vi "位置显示 ccd2.vi"(8 "error in (no error) 2":errorcluster, 10 "簇":T2, 11 "Image in":T1(plugin-control)) -> (0 "error out":errorcluster caption="错误输出", 1 "下":dbl, 2 "上":dbl, 3 "Image out":T1(plugin-control), 4 "x或y？":bool)   [LabVIEW 2017]
panel:
  out "xia":dbl
  out "shang":dbl
  out "x/y":dbl
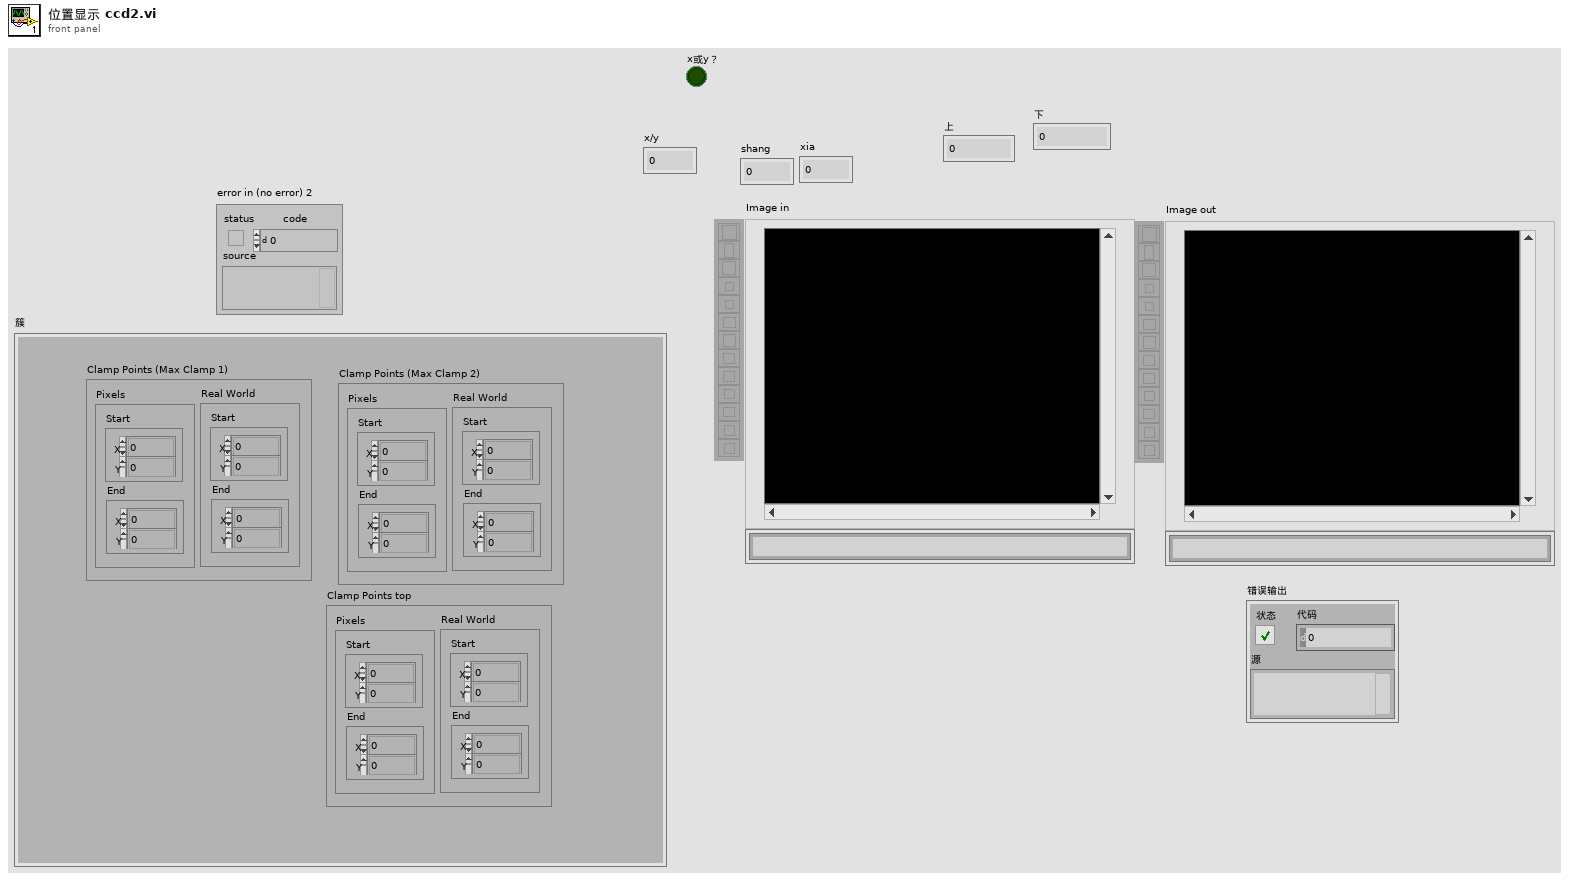
[diagram p1: front panel]
types:
  T1 = typedef "IMAQ Image.ctl" = refnum<image>
  T2 = cluster{"Clamp Points (Max Clamp 1)":cluster{"Pixels ":cluster{"Start":cluster{"X":dbl, "Y":dbl}, "End":cluster{"X":dbl, "Y":dbl}}, "Real World":cluster{"Start":cluster{"X":dbl, "Y":dbl}, "End":cluster{"X":dbl, "Y":dbl}}}, "Clamp Points (Max Clamp 2)":cluster{"Pixels ":cluster{"Start":cluster{"X":dbl, "Y":dbl}, "End":cluster{"X":dbl, "Y":dbl}}, "Real World":cluster{"Start":cluster{"X":dbl, "Y":dbl}, "End":cluster{"X":dbl, "Y":dbl}}}, "Clamp Points top":cluster{"Pixels ":cluster{"Start":cluster{"X":dbl, "Y":dbl}, "End":cluster{"X":dbl, "Y":dbl}}, "Real World":cluster{"Start":cluster{"X":dbl, "Y":dbl}, "End":cluster{"X":dbl, "Y":dbl}}}}
  T3 = cluster{"Pixels ":cluster{"Start":cluster{"X":dbl, "Y":dbl}, "End":cluster{"X":dbl, "Y":dbl}}, "Real World":cluster{"Start":cluster{"X":dbl, "Y":dbl}, "End":cluster{"X":dbl, "Y":dbl}}}
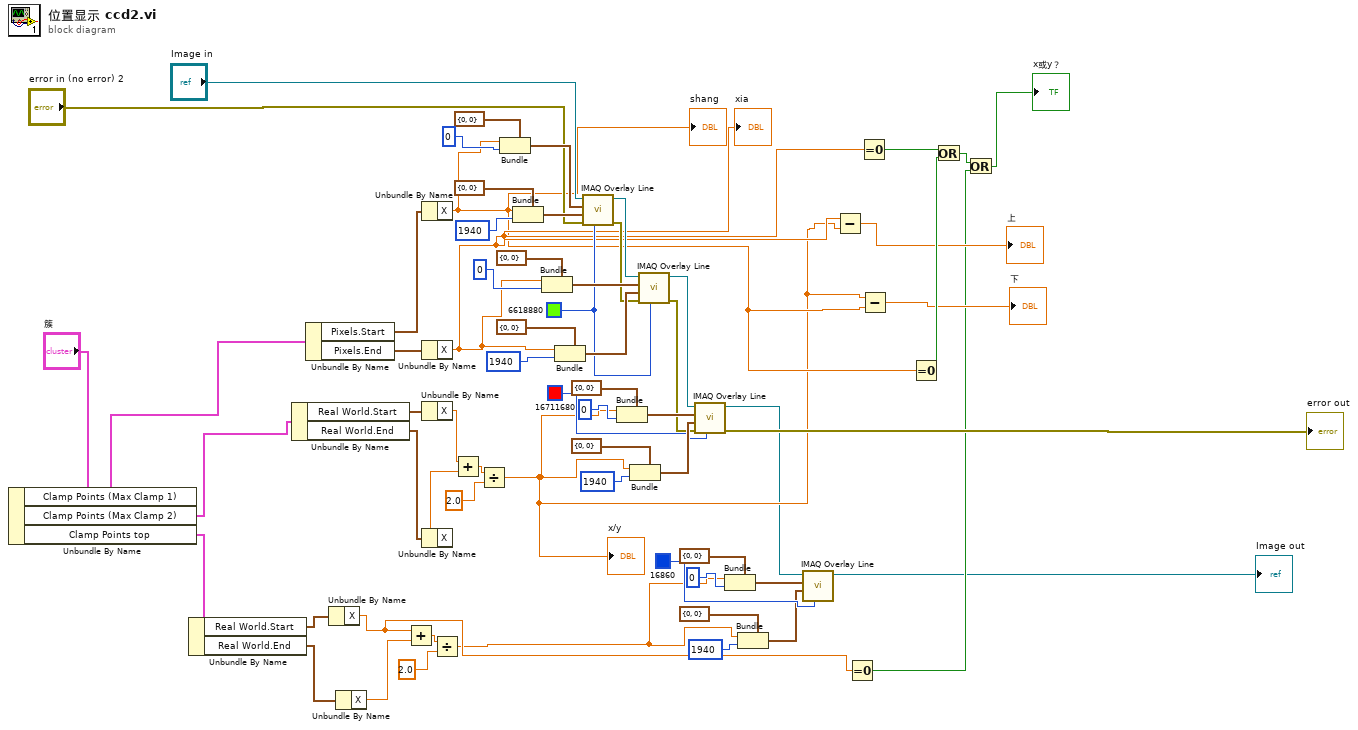
[diagram p0: block diagram]
diagram:
  w46 = u32 6618880 ("Color")
  n1 = Unbundle By Name("簇") -> ("Clamp Points (Max Clamp 1)"=w31:T3, "Clamp Points (Max Clamp 2)"=w30:T3, "Clamp Points top"=w21:T3)
  n2 = Unbundle By Name(w21) -> ("Real World.Start"=w20:cluster{"X":dbl, "Y":dbl}, "Real World.End"=w19:cluster{"X":dbl, "Y":dbl})
  n3 = Unbundle By Name(w30) -> ("Real World.Start"=w57:cluster{"X":dbl, "Y":dbl}, "Real World.End"=w54:cluster{"X":dbl, "Y":dbl})
  n4 = Unbundle By Name(w31) -> ("Pixels.Start"=w65:cluster{"X":dbl, "Y":dbl}, "Pixels.End"=w60:cluster{"X":dbl, "Y":dbl})
  n5 = Unbundle By Name(w20) -> ("X"=w15:dbl)
  n6 = Unbundle By Name(w19) -> ("X"=w16:dbl)
  n7 = Add(x=w15, y=w16) -> (x+y=w17:dbl)
  n8 = Unbundle By Name(w65) -> ("X"=w22:dbl)
  "shang" <- w22
  n9 = Unbundle By Name(w60) -> ("X"=w23:dbl)
  "xia" <- w23
  n10 = Unbundle By Name(w57) -> ("X"=w43:dbl)
  n11 = Unbundle By Name(w54) -> ("X"=w42:dbl)
  n12 = Divide(x=w17, y=2.0) -> (x/y=w3:dbl)
  n13 = Add(x=w43, y=w42) -> (x+y=w45:dbl)
  n14 = Divide(x=w45, y=2.0) -> (x/y=w11:dbl)
  "x/y" <- w11
  n15 = Bundle(cluster=cluster{"X":i32, "Y":i32} {"X"=0, "Y"=0} ("End Point"), "X"=w22, "Y"=0) -> (w52:cluster{"X":i32, "Y":i32})
  n16 = Bundle(cluster=cluster{"X":i32, "Y":i32} {"X"=0, "Y"=0} ("End Point"), "X"=w22, "Y"=1940) -> (w62:cluster{"X":i32, "Y":i32})
  n17 = Bundle(cluster=cluster{"X":i32, "Y":i32} {"X"=0, "Y"=0} ("End Point"), "X"=w23, "Y"=0) -> (w50:cluster{"X":i32, "Y":i32})
  n18 = Bundle(cluster=cluster{"X":i32, "Y":i32} {"X"=0, "Y"=0} ("End Point"), "X"=w23, "Y"=1940) -> (w58:cluster{"X":i32, "Y":i32})
  n19 = call "IMAQ Overlay Line"("Color"=w46, "error in (no error)"="error in (no error) 2", "End Point"=w62, "Start Point"=w52, "Image"="Image in") -> ("error out"=w35:errorcluster, "Image Out"=w61:T1)  [unwired: 5 in]
  n20 = Bundle(cluster=cluster{"X":i32, "Y":i32} {"X"=0, "Y"=0} ("End Point"), "X"=w11, "Y"=0) -> (w48:cluster{"X":i32, "Y":i32})
  n21 = Bundle(cluster=cluster{"X":i32, "Y":i32} {"X"=0, "Y"=0} ("End Point"), "X"=w11, "Y"=1940) -> (w56:cluster{"X":i32, "Y":i32})
  n22 = call "IMAQ Overlay Line"("Color"=w46, "error in (no error)"=w35, "End Point"=w58, "Start Point"=w50, "Image"=w61) -> ("error out"=w34:errorcluster, "Image Out"=w55:T1)  [unwired: 5 in]
  n23 = call "IMAQ Overlay Line"("Color"=u32 16711680, "error in (no error)"=w34, "End Point"=w56, "Start Point"=w48, "Image"=w55) -> ("error out"=→"error out":errorcluster, "Image Out"=w2:T1)  [unwired: 5 in]
  n24 = Bundle(cluster=cluster{"X":i32, "Y":i32} {"X"=0, "Y"=0} ("End Point"), "X"=w3, "Y"=0) -> (w7:cluster{"X":i32, "Y":i32})
  n25 = Bundle(cluster=cluster{"X":i32, "Y":i32} {"X"=0, "Y"=0} ("End Point"), "X"=w3, "Y"=1940) -> (w5:cluster{"X":i32, "Y":i32})
  n26 = call "IMAQ Overlay Line"("Color"=u32 16860, "End Point"=w5, "Start Point"=w7, "Image"=w2) -> ("Image Out"=→"Image out":T1)  [unwired: 6 in, 1 out]
  n27 = Subtract(x=w23, y=w11) -> (x-y=→"上":dbl)
  n28 = Equal To 0?(x=w15) -> (x = 0?=w13:bool)
  n29 = Equal To 0?(x=w23) -> (x = 0?=w41:bool)
  n30 = Subtract(x=w11, y=w22) -> (x-y=→"下":dbl)
  n31 = Equal To 0?(x=w22) -> (x = 0?=w40:bool)
  n32 = Or(x=w41, y=w40) -> (x .or. y?=w14:bool)
  n33 = Or(x=w14, y=w13) -> (x .or. y?=→"x或y？":bool)
